vi "dfd_Classical IIR Filters.vi"(4 "ripples [dB]":T2 {"stopband atten" format="%.2f"; "passband ripple" format="%.2f"}, 5 "filter design":T3(ring), 6 "fs [Hz]":dbl=1.0 format="%.2f", 7 "filter type":T1(ring), 9 "low cutoff freq: fl":dbl, 10 "high cutoff freq: fh":dbl, 11 "order":i32=2) -> (1 "poles":T4[](array[typedef]), 2 "zeros":T4[](array[typedef]), 3 "gain":dbl=1.0 format="%.4e")   [LabVIEW 2017, in "NI_DigFilter_Design.lvlib"]
doc: "Generates the poles and zeros of an IIR filter as specified by the filter model."
uses:
  <vilib>/addons/Digital Filter Design/NI_DigFilter_Design.lvlib
  <vilib>/addons/Digital Filter Design/_Objects.llb/DFD Pole-Zero.ctl
  <vilib>/addons/Digital Filter Design/NI_DigFilterLicensed.lvlib
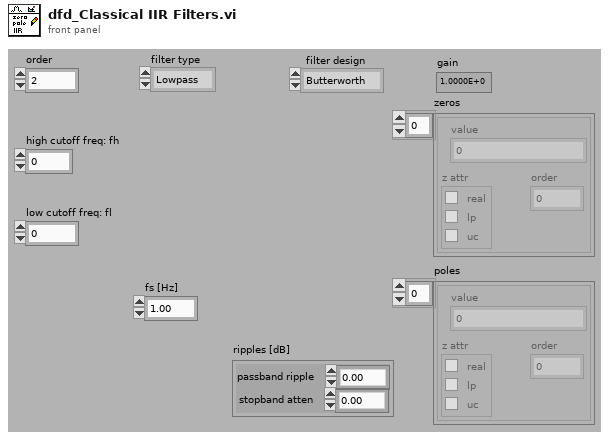
[diagram p1: front panel]
types:
  T1 = enum16{"Lowpass", "Highpass", "Bandpass", "Bandstop"}
  T2 = cluster{"passband ripple":dbl, "stopband atten":dbl}
  T3 = enum16{"Butterworth", "Chebyshev", "Inv Chebyshev", "Elliptic", "Bessel"}
  T4 = typedef "NI_DigFilterLicensed.lvlib/DFD Pole-Zero.ctl" = cluster{"value":cdb, "z attr":cluster{"real":bool, "lp":bool, "uc":bool}, "order":i32}
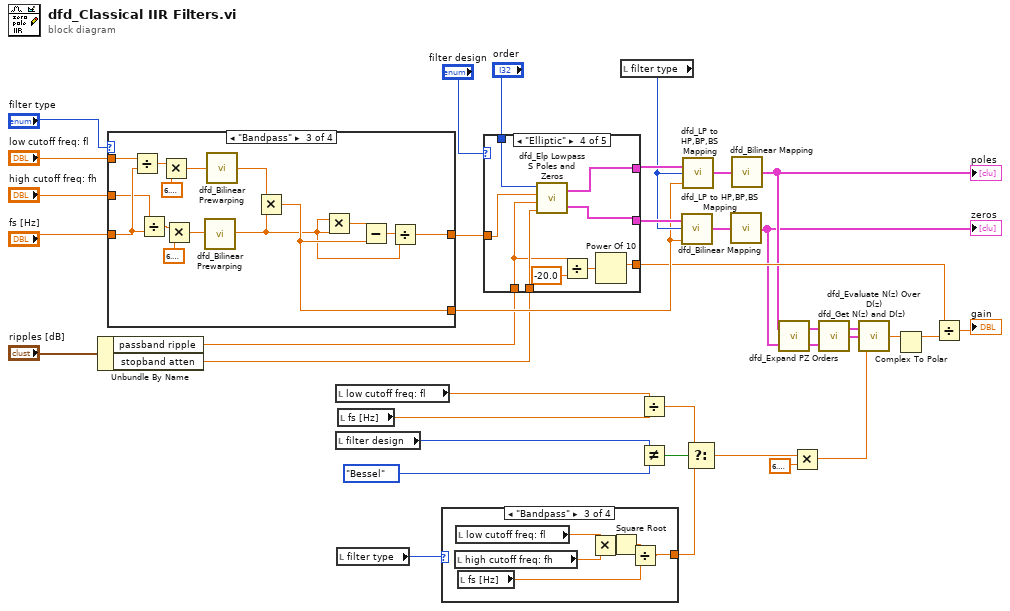
[diagram p0: block diagram]
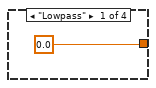
[diagram p2: hidden frame]
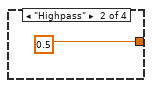
[diagram p3: hidden frame]
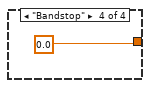
[diagram p4: hidden frame]
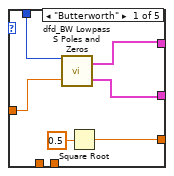
[diagram p5: hidden frame]
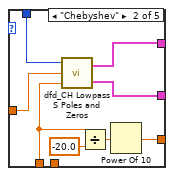
[diagram p6: hidden frame]
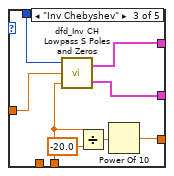
[diagram p7: hidden frame]
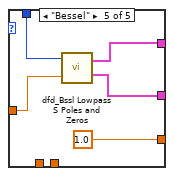
[diagram p8: hidden frame]
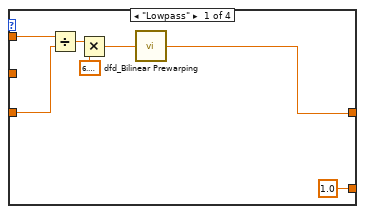
[diagram p9: hidden frame]
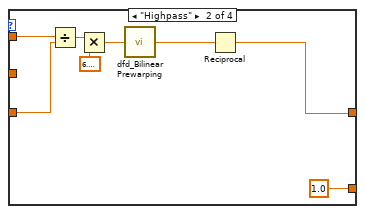
[diagram p10: hidden frame]
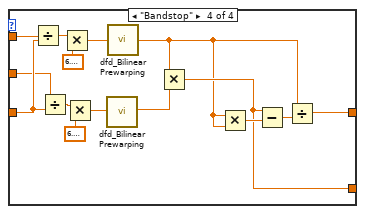
[diagram p11: hidden frame]
diagram:
  n1 = Unbundle By Name("ripples [dB]") -> ("passband ripple"=w7:dbl, "stopband atten"=w6:dbl)
  n2 = case shown="\"Bandpass\"" "filter type" {
    tunnel: "fs [Hz]" -> [w39 w47 w59 w76]
    tunnel: "low cutoff freq: fl" -> [w40 w48 w58 w75]
    tunnel: "high cutoff freq: fh" -> [_ _ w57 w74]
    tunnel: [w38 w45 w56 w72] -> w36
    tunnel: [1.0 1.0 w55 w69] -> w30
    frame "Lowpass" {
      n3 = Divide(x=w40, y=w39) -> (x/y=w41:dbl)
      n4 = Multiply(x=w41, y=6.283185307179586) -> (x*y=w43:dbl)
      n5 = call <vilib>:"dfd_Bilinear Prewarping.vi"("w"=w43) -> ("prewarped w"=w38:dbl)
    }
    frame "Highpass" {
      n6 = Divide(x=w48, y=w47) -> (x/y=w49:dbl)
      n7 = Multiply(x=w49, y=6.283185307179586) -> (x*y=w51:dbl)
      n8 = call <vilib>:"dfd_Bilinear Prewarping.vi"("w"=w51) -> ("prewarped w"=w46:dbl)
      n9 = Reciprocal(x=w46) -> (1/x=w45:dbl)
    }
    frame "Bandpass" {
      n10 = Divide(x=w58, y=w59) -> (x/y=w60:dbl)
      n11 = Divide(x=w57, y=w59) -> (x/y=w63:dbl)
      n12 = Multiply(x=w60, y=6.283185307179586) -> (x*y=w65:dbl)
      n13 = Multiply(x=w63, y=6.283185307179586) -> (x*y=w67:dbl)
      n14 = call <vilib>:"dfd_Bilinear Prewarping.vi"("w"=w67) -> ("prewarped w"=w53:dbl)
      n15 = call <vilib>:"dfd_Bilinear Prewarping.vi"("w"=w65) -> ("prewarped w"=w66:dbl)
      n16 = Multiply(x=w66, y=w53) -> (x*y=w55:dbl)
      n17 = Multiply(x=w53, y=w53) -> (x*y=w64:dbl)
      n18 = Subtract(x=w64, y=w55) -> (x-y=w54:dbl)
      n19 = Divide(x=w54, y=w53) -> (x/y=w56:dbl)
    }
    frame "Bandstop" {
      n20 = Divide(x=w75, y=w76) -> (x/y=w77:dbl)
      n21 = Divide(x=w74, y=w76) -> (x/y=w80:dbl)
      n22 = Multiply(x=w77, y=6.283185307179586) -> (x*y=w81:dbl)
      n23 = Multiply(x=w80, y=6.283185307179586) -> (x*y=w82:dbl)
      n24 = call <vilib>:"dfd_Bilinear Prewarping.vi"("w"=w82) -> ("prewarped w"=w71:dbl)
      n25 = call <vilib>:"dfd_Bilinear Prewarping.vi"("w"=w81) -> ("prewarped w"=w68:dbl)
      n26 = Multiply(x=w68, y=w71) -> (x*y=w69:dbl)
      n27 = Multiply(x=w68, y=w68) -> (x*y=w73:dbl)
      n28 = Subtract(x=w69, y=w73) -> (x-y=w70:dbl)
      n29 = Divide(x=w68, y=w70) -> (x/y=w72:dbl)
    }
  }
  n30 = local read "low cutoff freq: fl"() -> (w19:dbl)
  n31 = local read "filter design"() -> (w21:T3)
  n32 = local read "filter type"() -> (w14:T1)
  n33 = local read "fs [Hz]"() -> (w18:dbl)
  n34 = case shown="\"Bandpass\"" w14 {
    tunnel: [0.0 0.5 w86 0.0] -> w13
    frame "Lowpass" {
    }
    frame "Highpass" {
    }
    frame "Bandpass" {
      n35 = local read "high cutoff freq: fh"() -> (w89:dbl)
      n36 = local read "low cutoff freq: fl"() -> (w90:dbl)
      n37 = local read "fs [Hz]"() -> (w87:dbl)
      n38 = Multiply(x=w90, y=w89) -> (x*y=w88:dbl)
      n39 = Square Root(x=w88) -> (sqrt(x)=w85:dbl)
      n40 = Divide(x=w85, y=w87) -> (x/y=w86:dbl)
    }
    frame "Bandstop" {
    }
  }
  n41 = case shown="\"Elliptic\"" "filter design" {
    tunnel: "order" -> [w97 w105 w113 w122 w127]
    tunnel: w36 -> [w96 w104 w112 w121 w126]
    tunnel: w7 -> [_ w98 _ w115 _]
    tunnel: w6 -> [_ _ w106 w120 _]
    tunnel: [w95 w103 w111 w119 w125] -> w33
    tunnel: [w94 w102 w110 w118 w124] -> w32
    tunnel: [w92 w99 w107 w114 1.0] -> w23
    frame "Butterworth" {
      n42 = call <vilib>:"dfd_BW Lowpass S Poles and Zeros.vi"("low cutoff freq: wl"=w96, "order"=w97) -> ("zeros"=w94:T4[], "poles"=w95:T4[])
      n43 = Square Root(x=0.5) -> (sqrt(x)=w92:dbl)
    }
    frame "Chebyshev" {
      n44 = call <vilib>:"dfd_CH Lowpass S Poles and Zeros.vi"("ripple(dB)"=w98, "low cutoff freq: wl"=w104, "order"=w105) -> ("zeros"=w102:T4[], "poles"=w103:T4[])
      n45 = Divide(x=w98, y=-20.0) -> (x/y=w100:dbl)
      n46 = Power Of 10(x=w100) -> (10^x=w99:dbl)
    }
    frame "Inv Chebyshev" {
      n47 = call <vilib>:"dfd_Inv CH Lowpass S Poles and Zeros.vi"("attenuation (dB)"=w106, "low cutoff freq: wl"=w112, "order"=w113) -> ("zeros"=w110:T4[], "poles"=w111:T4[])
      n48 = Divide(x=w106, y=-20.0) -> (x/y=w108:dbl)
      n49 = Power Of 10(x=w108) -> (10^x=w107:dbl)
    }
    frame "Elliptic" {
      n50 = call <vilib>:"dfd_Elp Lowpass S Poles and Zeros.vi"("attenuation(dB)"=w120, "ripple(dB)"=w115, "low cutoff freq: wl"=w121, "order"=w122) -> ("zeros"=w118:T4[], "poles"=w119:T4[])
      n51 = Divide(x=w115, y=-20.0) -> (x/y=w116:dbl)
      n52 = Power Of 10(x=w116) -> (10^x=w114:dbl)
    }
    frame "Bessel" {
      n53 = call <vilib>:"dfd_Bssl Lowpass S Poles and Zeros.vi"("low cutoff freq: wl"=w126, "order"=w127) -> ("zeros"=w124:T4[], "poles"=w125:T4[])
    }
  }
  n54 = local read "filter type"() -> (w31:T1)
  n55 = Divide(x=w19, y=w18) -> (x/y=w16:dbl)
  n56 = Not Equal?(x=w21, y=T3."Bessel") -> (x != y?=w17:bool)
  n57 = call <vilib>:"dfd_LP to HP,BP,BS Mapping.vi"("wo^2"=w30, "filter type"=w31, "LP poles/zeros"=w32) -> ("transformed poles/zeros"=w34:T4[])
  n58 = call <vilib>:"dfd_LP to HP,BP,BS Mapping.vi"("wo^2"=w30, "filter type"=w31, "LP poles/zeros"=w33) -> ("transformed poles/zeros"=w35:T4[])
  n59 = Select(t=w16, s=w17, f=w13) -> (s? t:f=w15:dbl)
  n60 = call <vilib>:"dfd_Bilinear Mapping.vi"("s-plane poles/zeros"=w34) -> ("z-plane poles/zeros"=w11:T4[])
  "zeros" <- w11
  n61 = call <vilib>:"dfd_Bilinear Mapping.vi"("s-plane poles/zeros"=w35) -> ("z-plane poles/zeros"=w12:T4[])
  "poles" <- w12
  n62 = call <vilib>:"dfd_Expand PZ Orders.vi"("zeros"=w11, "poles"=w12) -> ("zeros expanded"=w9:T4[], "poles expanded"=w10:T4[])
  n63 = Multiply(x=w15, y=6.283185307179586) -> (x*y=w28:dbl)
  n64 = call <vilib>:"dfd_Get N(z) and D(z).vi"("zeros"=w9, "poles"=w10) -> ("D(z)"=w27:cluster{"Di(z)":dbl[]}[], "N(z)"=w26:cluster{"Ni(z)":dbl[]}[])
  n65 = call <vilib>:"dfd_Evaluate N(z) Over D(z).vi"("w"=w28, "D(z)"=w27, "N(z)"=w26) -> ("H(exp(jw))"=w25:cdb)
  n66 = Complex To Polar(r * e^(i*theta)=w25) -> (r=w24:dbl)  [unwired: 1 out]
  n67 = Divide(x=w23, y=w24) -> (x/y=→"gain":dbl)
